vi "Set Dyn Vars.vi"(8 "error in":errorcluster, 10 "Data":dbl, 11 "Set Values":T1) -> (0 "error out":errorcluster)   [LabVIEW 2014, in "CAN Bus Monitor Engine.lvlib"]
uses:
  CAN Bus Monitor Engine.lvlib
  Controls/Set Dyn Vars.ctl
  BM Global Vars.vi
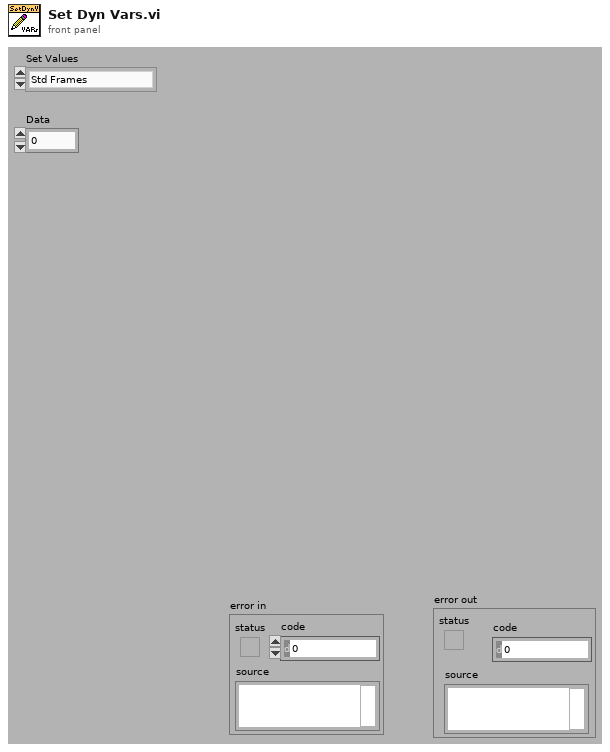
[diagram p1: front panel]
types:
  T1 = typedef "CAN Bus Monitor Engine.lvlib/Set Dyn Vars.ctl" = enum16{"Std Frames", "Std Frames / Sec", "Ext Frames", "Ext Frames / Sec", "Remote Frames", "Remote Frames / Sec", "Error Frames", "Error Frames / Sec", "BusLoad", "SumFrames", "SumFrames / Sec", "Null Frames", "Null Frames / Sec", "Peak Bus Load", "State", "IncMinFrameTime", "IncMaxFrameTime", "Driver Status", "CAN Comm State", "LIN Comm State", "FlexRay Comm State"}
  T2 = cluster{"IncMinFrameTime":dbl, "IncMaxFrameTime":dbl, "Min Frame Length":dbl[][], "Max Frame Length":dbl[][], "Std Frames":u32, "Ext Frames":u32, "Error Frames":u32, "Remote Frames":u32, "Std Frames / Sec":u32, "Ext Frames / Sec":u32, "Error Frames / Sec":u32, "Remote Frames / Sec":u32, "Peak Bus Load":dbl, "Bus Load":dbl, "Start Timestamp":dbl, "Null Frames":u32, "Null Frames / Sec":u32}
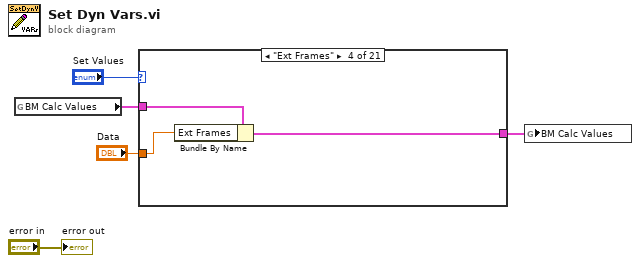
[diagram p0: block diagram]
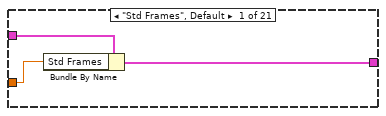
[diagram p2: hidden frame]
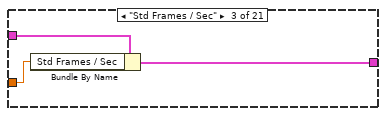
[diagram p4: hidden frame]
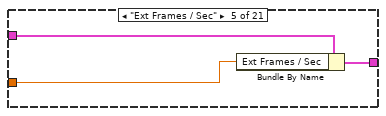
[diagram p5: hidden frame]
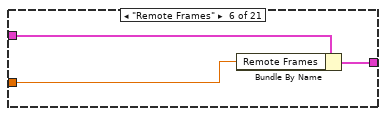
[diagram p6: hidden frame]
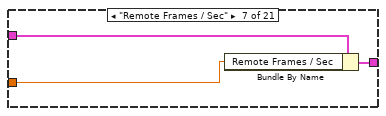
[diagram p7: hidden frame]
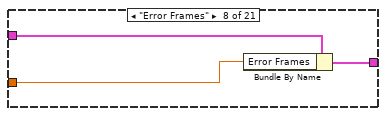
[diagram p8: hidden frame]
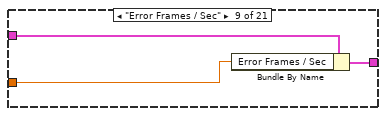
[diagram p9: hidden frame]
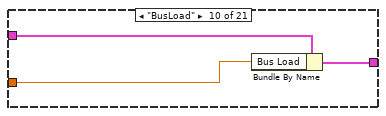
[diagram p10: hidden frame]
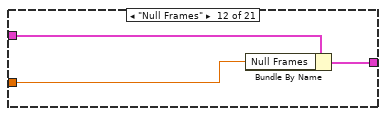
[diagram p12: hidden frame]
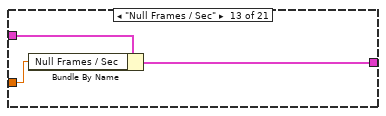
[diagram p13: hidden frame]
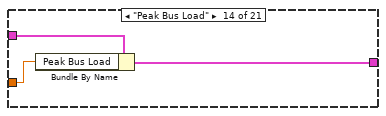
[diagram p14: hidden frame]
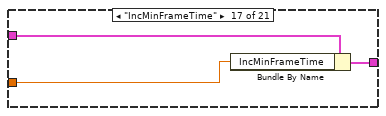
[diagram p17: hidden frame]
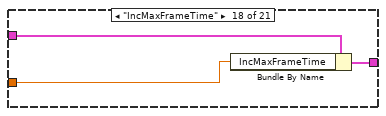
[diagram p18: hidden frame]
diagram:
  n1 = global read "BM Global Vars.vi" "BM Calc Values"() -> (w4:T2)
  n2 = case shown="\"Ext Frames\"" "Set Values" {
    tunnel: w4 -> [w7 w9 w12 w15 w16 w21 w24 w25 w29 w31 w34 w35 w40 w43 w44 w45 w47 w51 w52 w53 w54]
    tunnel: [w6 w9 w11 w14 w17 w20 w23 w26 w28 w33 w34 w37 w39 w42 w44 w45 w46 w50 w52 w53 w54] -> w3
    tunnel: "Data" -> [w8 _ w10 w13 w18 w19 w22 w27 w30 w32 _ w36 w38 w41 _ _ w48 w49 _ _ _]
    frame "Std Frames", Default {
      n3 = Bundle By Name(cluster=w7, "Std Frames"=w8) -> (w6:T2)
    }
    frame "Driver Status" {
    }
    frame "Std Frames / Sec" {
      n4 = Bundle By Name(cluster=w12, "Std Frames / Sec"=w10) -> (w11:T2)
    }
    frame "Ext Frames" {
      n5 = Bundle By Name(cluster=w15, "Ext Frames"=w13) -> (w14:T2)
    }
    frame "Ext Frames / Sec" {
      n6 = Bundle By Name(cluster=w16, "Ext Frames / Sec"=w18) -> (w17:T2)
    }
    frame "Remote Frames" {
      n7 = Bundle By Name(cluster=w21, "Remote Frames"=w19) -> (w20:T2)
    }
    frame "Remote Frames / Sec" {
      n8 = Bundle By Name(cluster=w24, "Remote Frames / Sec"=w22) -> (w23:T2)
    }
    frame "Error Frames" {
      n9 = Bundle By Name(cluster=w25, "Error Frames"=w27) -> (w26:T2)
    }
    frame "Error Frames / Sec" {
      n10 = Bundle By Name(cluster=w29, "Error Frames / Sec"=w30) -> (w28:T2)
    }
    frame "BusLoad" {
      n11 = Bundle By Name(cluster=w31, "Bus Load"=w32) -> (w33:T2)
    }
    frame "SumFrames" {
    }
    frame "Null Frames" {
      n12 = Bundle By Name(cluster=w35, "Null Frames"=w36) -> (w37:T2)
    }
    frame "Null Frames / Sec" {
      n13 = Bundle By Name(cluster=w40, "Null Frames / Sec"=w38) -> (w39:T2)
    }
    frame "Peak Bus Load" {
      n14 = Bundle By Name(cluster=w43, "Peak Bus Load"=w41) -> (w42:T2)
    }
    frame "State" {
    }
    frame "SumFrames / Sec" {
    }
    frame "IncMinFrameTime" {
      n15 = Bundle By Name(cluster=w47, "IncMinFrameTime"=w48) -> (w46:T2)
    }
    frame "IncMaxFrameTime" {
      n16 = Bundle By Name(cluster=w51, "IncMaxFrameTime"=w49) -> (w50:T2)
    }
    frame "CAN Comm State" {
    }
    frame "LIN Comm State" {
    }
    frame "FlexRay Comm State" {
    }
  }
  n17 = global write "BM Global Vars.vi" "BM Calc Values"(w3) -> ()
  "error out" <- "error in"
